vi "Filter Exclusions.vi"(10 "Group Names":string[](array[string])) -> (2 "Group Names Out":string[](array[string]))   [LabVIEW 2013]
panel:
  in  "Keep Root":bool[](array[boolean])=[TRUE, FALSE]
  in  "Exclusions":string[](array[string])=["External/", "Consolidated/Act/"]
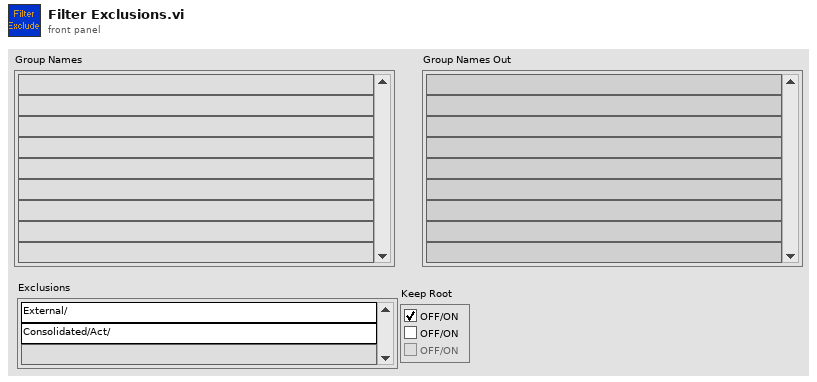
[diagram p1: front panel]
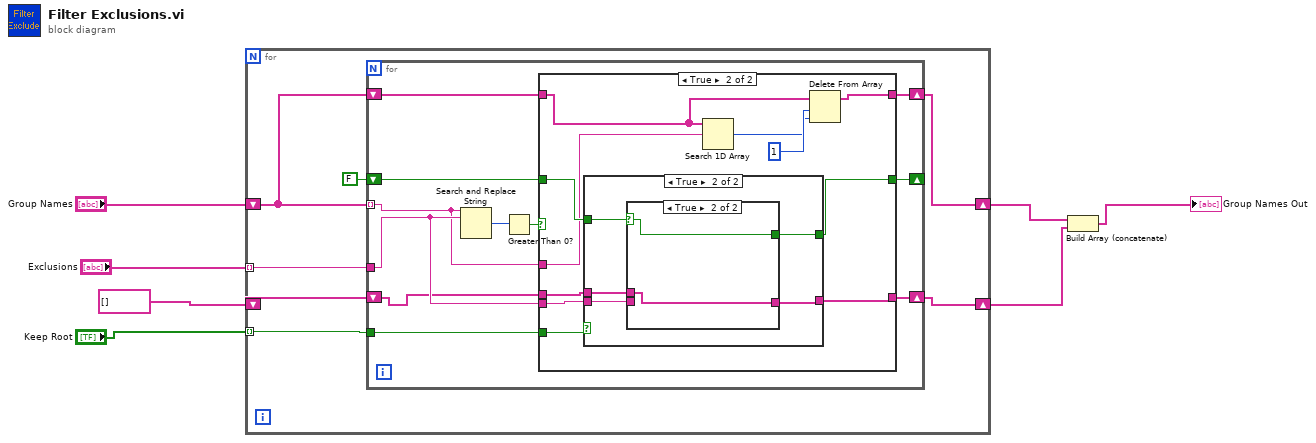
[diagram p0: block diagram]
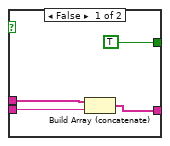
[diagram p4: hidden frame]
diagram:
  n1 = for {
    tunnel: "Exclusions" -> [w14] mode=indexing
    tunnel: "Keep Root" -> [w13] mode=indexing
    shift-right: [w10] -> w4
    shift-left: "Group Names" -> [w11]
    shift-right: [w9] -> w3
    shift-left: string[] [] -> [w8]
    n2 = for {
      tunnel: w11 -> [w19] mode=indexing
      tunnel: w14 -> [w21]
      tunnel: w13 -> [w23]
      shift-right: [w20] -> _
      shift-left: FALSE -> [w22]
      shift-right: [w17] -> w10
      shift-left: w11 -> [w18]
      shift-right: [w16] -> w9
      shift-left: w8 -> [w15]
      n3 = Search and Replace String(input string=w19, search string=w21) -> (number of replacements=w25:i32)  [unwired: 6 in, 3 out]
      n4 = Greater Than 0?(x=w25) -> (x > 0?=w24:bool)
      n5 = case shown="True" w24 {
        tunnel: w23 -> [_ w39]
        tunnel: w22 -> [w28 w38]
        tunnel: w21 -> [_ w37]
        tunnel: w15 -> [w26 w34]
        tunnel: [w28 w36] -> w20
        tunnel: w19 -> [_ w30]
        tunnel: w18 -> [w27 w31]
        tunnel: [w27 w32] -> w17
        tunnel: [w26 w33] -> w16
        frame False {
        }
        frame True {
          n6 = case shown="True" w39 {
            tunnel: w38 -> [w41 w46]
            tunnel: w37 -> [_ w45]
            tunnel: w34 -> [w40 w44]
            tunnel: [w41 w43] -> w36
            tunnel: [w40 w42] -> w33
            frame False {
            }
            frame True {
              n7 = case shown="True" w46 {
                selector: w46 -> [_ w52]
                tunnel: w45 -> [w50 _]
                tunnel: [w49 w51] -> w42
                tunnel: w44 -> [w48 w51]
                tunnel: [TRUE w52] -> w43
                frame False {
                  n8 = Build Array (concatenate)(w48, w50) -> (w49:string[])
                }
                frame True {
                }
              }
            }
          }
          n9 = Search 1D Array(1D array=w31, element=w30) -> (index of element=w29:i32)  [unwired: 1 in]
          n10 = Delete From Array(array=w31, length=1, index=w29) -> (array with subset deleted=w32:string[])  [unwired: 1 out]
        }
      }
    }
  }
  n11 = Build Array (concatenate)(w4, w3) -> (→"Group Names Out":string[])
